vi "Add Error Status Channels.vi"(8 "error in":errorcluster, 11 "status section ref":T1 format="%.0x") -> (0 "error out":errorcluster, 3 "status section ref out":T1 format="%.0x")   [LabVIEW 2020, in "Ballard ARINC 429 Scripting.lvlib"]
uses:
  Ballard ARINC 429 Scripting.lvlib
  <vilib>/NI VeriStand/Custom Device API/Custom Device Item Ref.ctl
  <vilib>/NI VeriStand/Custom Device API/Custom Device Channel.ctl
  <vilib>/NI VeriStand/Custom Device API/Custom Device Channel Type.ctl
  Constants.vi
  <vilib>/NI VeriStand/Custom Device API/Custom Device API.lvlib
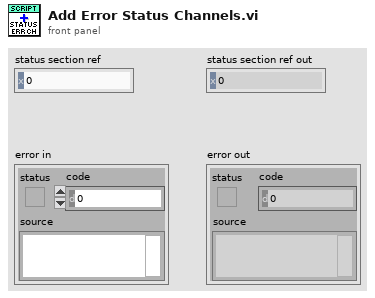
[diagram p1: front panel]
types:
  T1 = typedef "Custom Device API.lvlib/Custom Device Item Ref.ctl" = u64
  T2 = typedef "Custom Device API.lvlib/Custom Device Channel.ctl" = cluster{"Type":T3, "Units":string, "Default Value":dbl, "Faultable":bool, "Scalable":bool}
  T3 = typedef "Custom Device API.lvlib/Custom Device Channel Type.ctl" = enum16{"Input", "Output"}
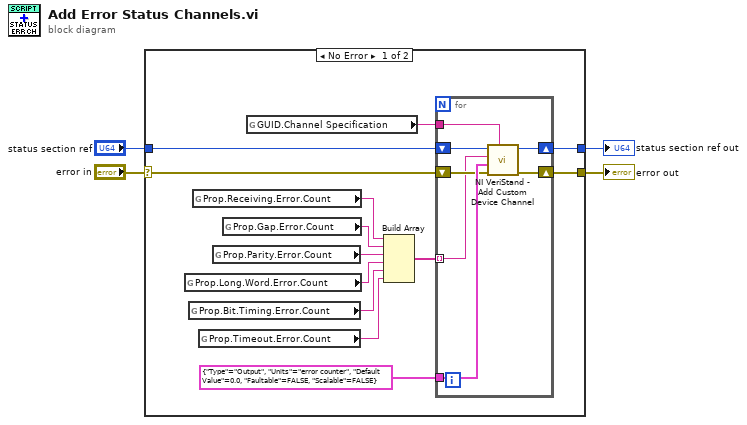
[diagram p0: block diagram]
diagram:
  n1 = case shown="No Error" "error in" {
    selector: "error in" -> [w17 w26]
    tunnel: "status section ref" -> [w16 w25]
    tunnel: [w13 w26] -> w3
    tunnel: [w12 w25] -> w2
    frame No Error {
      n2 = global read "Constants.vi" "Prop.Long.Word.Error.Count"() -> (w7:string)
      n3 = global read "Constants.vi" "Prop.Bit.Timing.Error.Count"() -> (w8:string)
      n4 = global read "Constants.vi" "Prop.Receiving.Error.Count"() -> (w11:string)
      n5 = global read "Constants.vi" "Prop.Timeout.Error.Count"() -> (w6:string)
      n6 = global read "Constants.vi" "Prop.Parity.Error.Count"() -> (w9:string)
      n7 = global read "Constants.vi" "Prop.Gap.Error.Count"() -> (w10:string)
      n8 = global read "Constants.vi" "GUID.Channel Specification"() -> (w15:string)
      n9 = Build Array(w11, w10, w9, w7, w8, w6) -> (w5:string[])
      n10 = for {
        tunnel: w15 -> [w23]
        tunnel: T2 {"Type"=enum."Output", "Units"="error counter", "Default Value"=0.0, "Faultable"=FALSE, "Scalable"=FALSE} ("Channel") -> [w22]
        shift-right: [w19] -> w12
        shift-left: w16 -> [w24]
        shift-right: [w20] -> w13
        shift-left: w17 -> [w21]
        tunnel: w5 -> [w18] mode=indexing
        n11 = call <vilib>:"NI VeriStand - Add Custom Device Channel.vi"("GUID (Default Channel)"=w23, "error in (no error)"=w21, "Channel"=w22, "Channel Name"=w18, "Parent Ref in"=w24) -> ("error out"=w20:errorcluster, "Parent Ref out"=w19:T1)  [unwired: 3 in, 2 out]
      }
    }
    frame Error {
    }
  }
  "error out" <- w3
  "status section ref out" <- w2
